vi "ramp trajectory.vi"(8 "points":i32=1000, 10 "end (volts)":sgl format="%.2f", 11 "start (volts)":sgl format="%.2f") -> (3 "ramp":sgl[](array[numeric]) format="%.2f")   [LabVIEW 2010]
uses:
  <vilib>/Analysis/NI_AALBase.lvlib
panel:
  out "?":dbl[](graph)
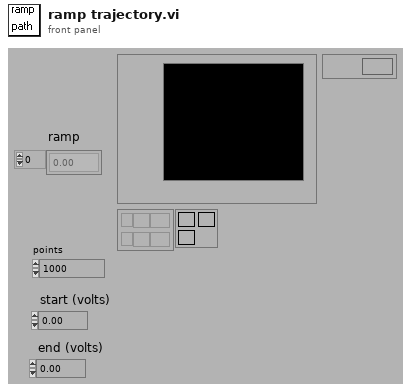
[diagram p1: front panel]
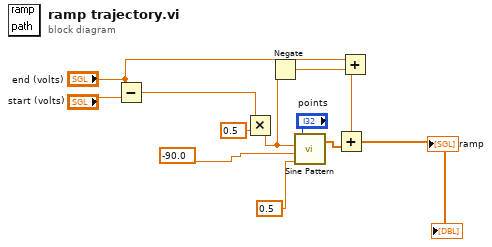
[diagram p0: block diagram]
diagram:
  n1 = Subtract(x="end (volts)", y="start (volts)") -> (x-y=w2:sgl)
  n2 = Multiply(x=w2, y=sgl 0.5) -> (x*y=w5:sgl)
  n3 = Negate(x=w5) -> (-x=w3:sgl)
  n4 = call <vilib>:"Sine Pattern.vi"("cycles"=0.5, "phase(degrees)"=-90.0, "amplitude"=w5, "samples"="points") -> ("Sinusoidal Pattern"=w9:dbl[])  [unwired: 1 out]
  n5 = Add(x="end (volts)", y=w3) -> (x+y=w4:sgl)
  n6 = Add(x=w4, y=w9) -> (x+y=→"ramp" →"?":dbl[])
